vi "Get Tx Hardware Channel Data.vi"(8 "error in":errorcluster, 11 "custom device ref in":T1 format="%.0x") -> (0 "error out":errorcluster, 1 "Tx hardware channel data":T2[](array[typedef]) {"labels settings for RT"."Label Timestamp Channel Data Reference" format="%.0x"; "labels settings for RT"."Word Initial Raw Value" format="%032.0f"; "labels settings for RT"."Label Disable/Trigger Channel Reference" format="%.0x"; "labels settings for RT"."parameter driver data"."Tx parameter refs" format="%.0x"; "labels settings for RT"."SDI" format="%02b"; "labels settings for RT"."label" format="%.0o"}, 2 "outgoing channels":T1[](array[typedef]) format="%.0x", 3 "custom device ref out":T1 format="%.0x")   [LabVIEW 2020]
uses:
  <vilib>/NI VeriStand/Custom Device API/Custom Device Item Ref.ctl
  RT Hardware Channel Settings.ctl
  RT Label Settings.ctl
  Label.ctl
  RT Parameters.ctl
  Parameter Definition.ctl
  <vilib>/addons/VeriStand Custom Device Scripting APIs/Ballard ARINC 429/Encoding and Decoding/Encoding.ctl
  Transfer Type.ctl
  <vilib>/NI VeriStand/Custom Device API/Data Reference.ctl
  Scripting/Ballard/Ballard ARINC 429 Scripting.lvlib
  <vilib>/NI VeriStand/Custom Device API/Custom Device API.lvlib
  <vilib>/addons/VeriStand Custom Device Scripting APIs/Ballard ARINC 429/Encoding and Decoding/Encoding and Decoding.lvlib
  Scripting/ARINC 429/ARINC 429 Scripting.lvlib
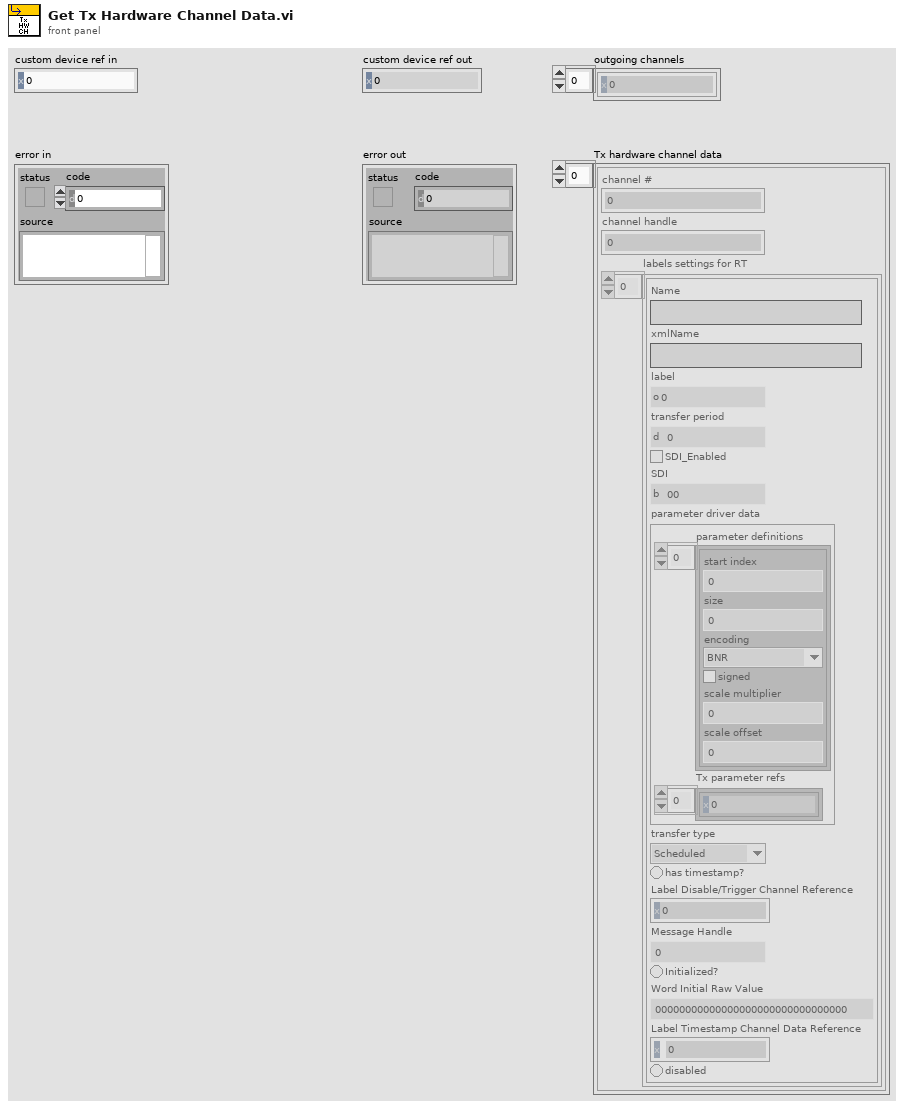
[diagram p1: front panel]
types:
  T1 = typedef "Custom Device API.lvlib/Custom Device Item Ref.ctl" = u64
  T2 = typedef "RT Hardware Channel Settings.ctl" = cluster{"channel #":u16, "channel handle":u64, "labels settings for RT":T3[]}
  T3 = typedef "RT Label Settings.ctl" = cluster{"Name":string, "xmlName":string, "label":T4, "transfer period":u32, "SDI_Enabled":bool, "SDI":u8, "parameter driver data":T5, "transfer type":T8, "has timestamp?":bool, "Label Disable/Trigger Channel Reference":T1, "Message Handle":u64, "Initialized?":bool, "Word Initial Raw Value":u32, "Label Timestamp Channel Data Reference":T9, "disabled":bool}
  T4 = typedef "Label.ctl" = u8
  T5 = typedef "RT Parameters.ctl" = cluster{"parameter definitions":T6[], "Tx parameter refs":T1[]}
  T6 = typedef "Parameter Definition.ctl" = cluster{"start index":i32, "size":i32, "encoding":T7, "signed":bool, "scale multiplier":dbl, "scale offset":dbl}
  T7 = typedef "Encoding and Decoding.lvlib/Encoding.ctl" = enum16{"BNR", "BCD", "Discrete"}
  T8 = typedef "Transfer Type.ctl" = enum16{"Scheduled", "Acyclic", "Block", "Strobe"}
  T9 = typedef "Custom Device API.lvlib/Data Reference.ctl" = i32
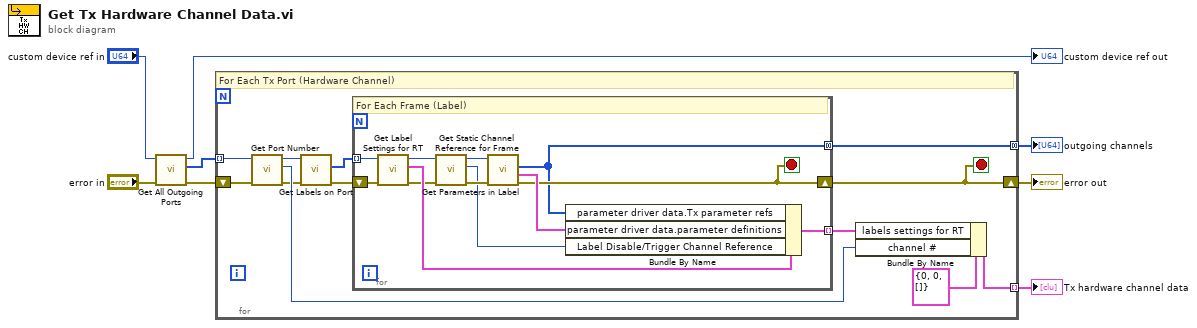
[diagram p0: block diagram]
diagram:
  n1 = call "Get All Outgoing Ports.vi"("error in"="error in", "Ballard ARINC 429 custom device in"="custom device ref in") -> ("error out"=w5:errorcluster, "outgoing ports"=w4:T1[], "Ballard ARINC 429 custom device out"=→"custom device ref out":T1)  [unwired: 7 in]
  n2 = for {
    shift-right: [w20] -> w7
    shift-left: w5 -> [w15]
    tunnel: w4 -> [w16] mode=indexing
    tunnel: [w19] -> w6 mode=indexing
    tunnel: [w9] -> w1 mode=concatenating
    stop <- w20 stop-if-true
    # "For Each Tx Port (Hardware Channel)"
    n3 = call "Get Port Number.vi"("error in"=w15, "port ref in"=w16) -> ("error out"=w12:errorcluster, "port number"=w14:u16, "port ref out"=w13:T1)  [unwired: 6 in, 1 out]
    n4 = call "Get Labels on Port.vi"("error in"=w12, "port in"=w13) -> ("error out"=w10:errorcluster, "labels"=w11:T1[])  [unwired: 6 in, 2 out]
    n5 = for {
      tunnel: w11 -> [w32] mode=indexing
      shift-right: [w23] -> w20
      shift-left: w10 -> [w31]
      tunnel: [w28] -> w18 mode=indexing
      tunnel: [w21] -> w9 mode=concatenating
      stop <- w23 stop-if-true
      # "For Each Frame (Label)"
      n6 = call "Get Label Settings for RT.vi"("error in"=w31, "label ref in"=w32) -> ("error out"=w27:errorcluster, "label settings for RT"=w30:T3, "label ref out"=w26:T1)  [unwired: 7 in]
      n7 = call "Get Static Channel Reference for Frame.vi"("error in"=w27, "label ref"=w26) -> ("error out"=w25:errorcluster, "channel specification ref"=w24:T1, "label ref out"=w22:T1)  [unwired: 6 in, 1 out]
      n8 = call "Get Parameters in Label.vi"("error in"=w25, "label in"=w22) -> ("error out"=w23:errorcluster, "parameter definitions"=w29:T6[], "parameters"=w21:T1[])  [unwired: 6 in, 1 out]
      n9 = Bundle By Name(cluster=w30, "parameter driver data.Tx parameter refs"=w21, "parameter driver data.parameter definitions"=w29, "Label Disable/Trigger Channel Reference"=w24) -> (w28:T3)
    }
    n10 = Bundle By Name(cluster=T2 {"channel #"=0, "channel handle"=0, "labels settings for RT"=[]} ("RT hardware channel"), "labels settings for RT"=w18, "channel #"=w14) -> (w19:T2)
  }
  "error out" <- w7
  "Tx hardware channel data" <- w6
  "outgoing channels" <- w1
